vi "Myrio_8.vi"() -> ()   [LabVIEW 2012]
uses:
  SubVIs/LVPresent_Globals.vi
panel:
  in  "Hint/Solution 4":bool
  in  "Hint/Solution 3":bool
  in  "Hint/Solution 2":bool
  in  "Hint/Solution":bool
  # "Hints"
  # "Hint 1: Start with a write command, because you will  want the light to output information. Also the first LED is of pin 13.Remember, if you need help, check out the menu in the bottom left corner."
  # "Hint 2: You will have to use a wait function."
  # "Hint 3: One case will require a For Loop; the other, a While Loop"
  # "Helpful Tip: When creating a constant, you can right click on the terminal and click creat-->constant. Note that constants are not always numbers."
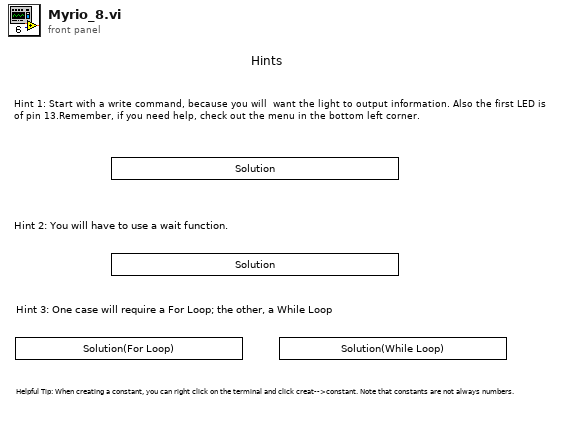
[diagram p1: front panel]
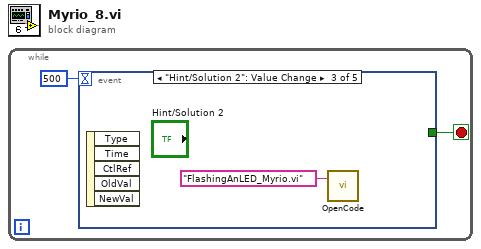
[diagram p0: block diagram]
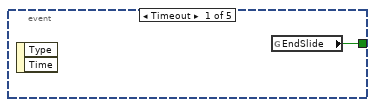
[diagram p2: hidden frame]
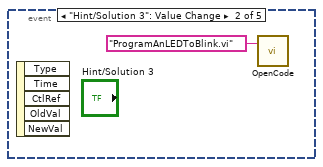
[diagram p3: hidden frame]
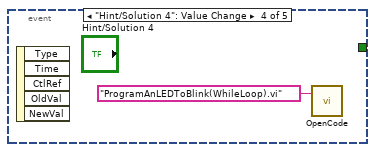
[diagram p4: hidden frame]
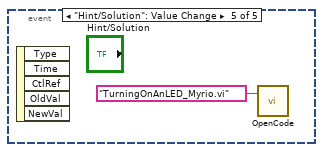
[diagram p5: hidden frame]
diagram:
  n1 = while {
    stop <- w2 stop-if-true
    n2 = event shown="[2] \"Hint/Solution 2\": Value Change" {
      selector: _ -> [_ _ _ _ _]
      dyn-events: _ -> [_ _ _ _ _]
      timeout: 500 -> [_ _ _ _ _]
      tunnel: [w3 _ _ _ _] -> w2
      event Timeout {
        n3 = event-data() -> ()  [unwired: 1 in, 2 out]
        n4 = global read "LVPresent_Globals.vi" "EndSlide"() -> (w3:bool)
      }
      event "Hint/Solution 3": Value Change {
        n5 = event-data() -> ()  [unwired: 1 in, 5 out]
        n6 = call "OpenCode.vi"("Code name"="ProgramAnLEDToBlink.vi") -> ()  [unwired: 3 in]
      }
      event "Hint/Solution 2": Value Change {
        n7 = event-data() -> ()  [unwired: 1 in, 5 out]
        n8 = call "OpenCode.vi"("Code name"="FlashingAnLED_Myrio.vi") -> ()  [unwired: 3 in]
      }
      event "Hint/Solution 4": Value Change {
        n9 = event-data() -> ()  [unwired: 1 in, 5 out]
        n10 = call "OpenCode.vi"("Code name"="ProgramAnLEDToBlink(WhileLoop).vi") -> ()  [unwired: 3 in]
      }
      event "Hint/Solution": Value Change {
        n11 = event-data() -> ()  [unwired: 1 in, 5 out]
        n12 = call "OpenCode.vi"("Code name"="TurningOnAnLED_Myrio.vi") -> ()  [unwired: 3 in]
      }
    }
  }
